vi "step function.vi"(1 "数值":i32) -> (0 "数值 2":i32)   [LabVIEW 2012]
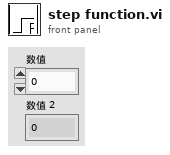
[diagram p1: front panel]
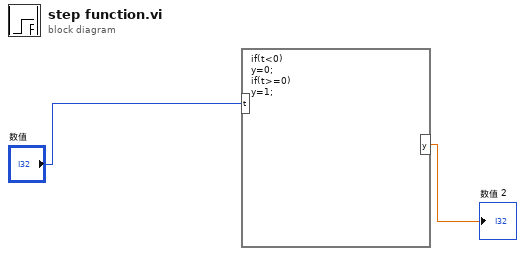
[diagram p0: block diagram]
diagram:
  n1 = formula code="if(t<0)\ny=0;\nif(t>=0)\ny=1;"("t"="数值") -> ("y"=→"数值 2":dbl)
